vi "MC get remote commands.vi"(11 "UDP Network Connection in":refnum<k16>) -> ()   [LabVIEW 2020]
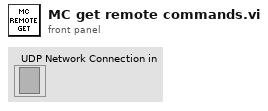
[diagram p1: front panel]
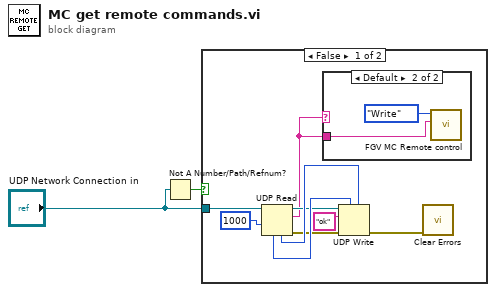
[diagram p0: block diagram]
diagram:
  n1 = Not A Number/Path/Refnum?(number/path/refnum="UDP Network Connection in") -> (NaN/Path/Refnum?=w1:bool)
  n2 = case shown="False" w1 {
    tunnel: "UDP Network Connection in" -> [w11 _]
    frame False {
      n3 = UDP Read(connection ID=w11, timeout ms (25000)=1000) -> (data out=w3:string, error out=w5:errorcluster, 3:w6:refnum<k16>, 4:w9:u16, 6:w8:u32)  [unwired: 2 in]
      n4 = case shown="Default" w3 {
        tunnel: w3 -> [_ w13]
        frame "\u0000" {
        }
        frame Default {
          n5 = call "FGV MC Remote control.vi"("slow response in"=w13, "Function"=enum16{"Read", "Write", "Clear"}."Write") -> ()  [unwired: 8 in, 2 out]
        }
      }
      n6 = UDP Write(address=w8, port or service name=w9, connection ID=w6, data in="ok", 8:w5) -> (error out=w4:errorcluster)  [unwired: 1 in, 1 out]
      n7 = call <vilib>:"Clear Errors.vi"("error in (no error)"=w4) -> ()  [unwired: 5 in, 2 out]
    }
    frame True {
    }
  }
